vi "WinCI NoOp.vi"(8 "error in (no error)":errorcluster) -> (0 "error out":errorcluster)   [LabVIEW 2020, in "NI_SCC_WinCI.lvlib"]
uses:
  <vilib>/SourceControl/Providers/WinCI/NI_SCC_WinCI.lvlib
  <vilib>/SourceControl/Providers/WinCI/WinCI Close Project.vi
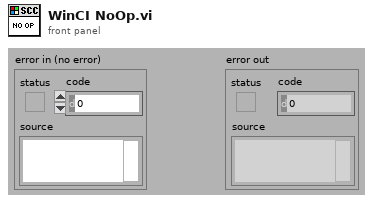
[diagram p1: front panel]
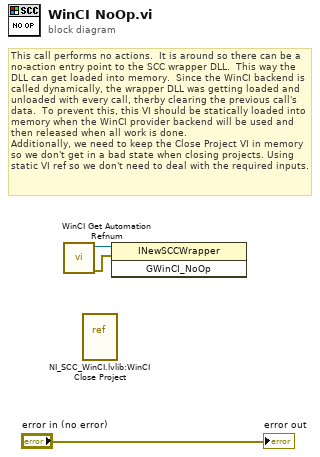
[diagram p0: block diagram]
diagram:
  # "This call performs no actions.  It is around so there can be a no-action entry point to the SCC wrapper DLL.  This way the DLL can get loaded into memory.  Since the WinCI backend is called dynamically, the wrapper DLL was getting loaded and unloaded with every call, therby clearing the previous call's data.  To prevent this, this VI should be statically loaded into memory when the WinCI provider backend will be used and then released when all work is done.\nAdditionally, we need to keep the Close Project VI in memory so we don't get in a bad state when closing projects. Using static VI ref so we don't need to deal with the required inputs."
  n1 = call <vilib>:"WinCI Get Automation Refnum.vi"() -> ("error out"=w2:errorcluster, "automation refnum"=w1:refnum<k7>)  [unwired: 10 out]
  n2 = vi-ref "NI_SCC_WinCI.lvlib:WinCI Close Project.vi"() -> ()  [unwired: 1 out]
  n3 = invoke class="INewSCCWrapper" method="GWinCI_NoOp"(reference=w1, error in=w2) -> ()  [unwired: 1 in, 3 out]
  "error out" <- "error in (no error)"
